vi "Nudge Rectangle.vi"(8 "error in (no error)":errorcluster, 9 "dy":i32, 10 "dx":i32, 11 "Rectangle":T1 {"Rotation" min=-90.0 max=90.0 step=1.0 format="%.2f"; "Left" scale=0.0..1024.0; "Right" scale=0.0..1024.0}) -> (0 "error out":errorcluster, 3 "Nudged Rectangle":T1 {"Rotation" min=-90.0 max=90.0 step=1.0 format="%.2f"; "Left" scale=0.0..1024.0; "Right" scale=0.0..1024.0})   [LabVIEW 2013]
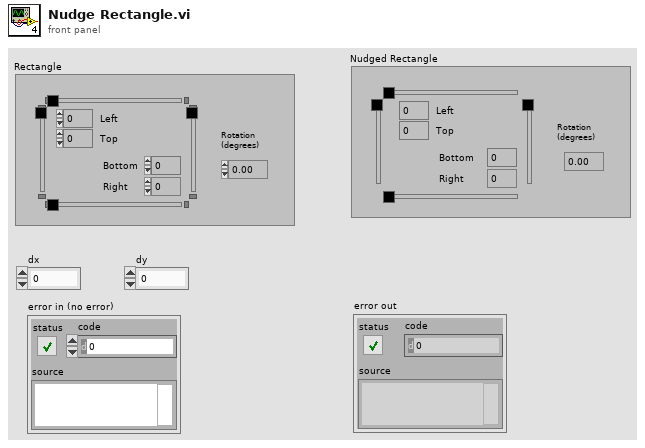
[diagram p1: front panel]
types:
  T1 = typedef "IMAQ Rectangle" = cluster{"Left":i32, "Top":i32, "Right":i32, "Bottom":i32, "Rotation":dbl}
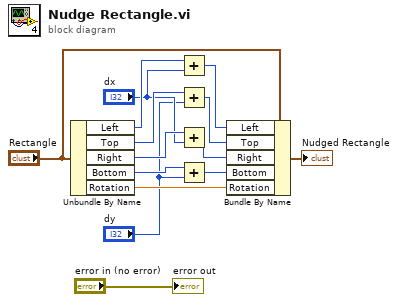
[diagram p0: block diagram]
diagram:
  n1 = Unbundle By Name("Rectangle") -> ("Left"=w11:i32, "Top"=w9:i32, "Right"=w7:i32, "Bottom"=w4:i32, "Rotation"=w13:dbl)
  n2 = Add(x=w11, y="dx") -> (x+y=w10:i32)
  n3 = Add(x=w9, y="dy") -> (x+y=w8:i32)
  n4 = Add(x=w7, y="dx") -> (x+y=w5:i32)
  n5 = Add(x=w4, y="dy") -> (x+y=w2:i32)
  n6 = Bundle By Name(cluster="Rectangle", "Left"=w10, "Top"=w8, "Right"=w5, "Bottom"=w2, "Rotation"=w13) -> (→"Nudged Rectangle":T1)
  "error out" <- "error in (no error)"
